vi "_PC_Spectrafilter get_tree_filter_data.vi"(8 "error in (no error)":errorcluster, 11 "file tree ref":refnum<vi>) -> (0 "error out":errorcluster, 2 "datas path":path[](array[path]))   [LabVIEW 2018]
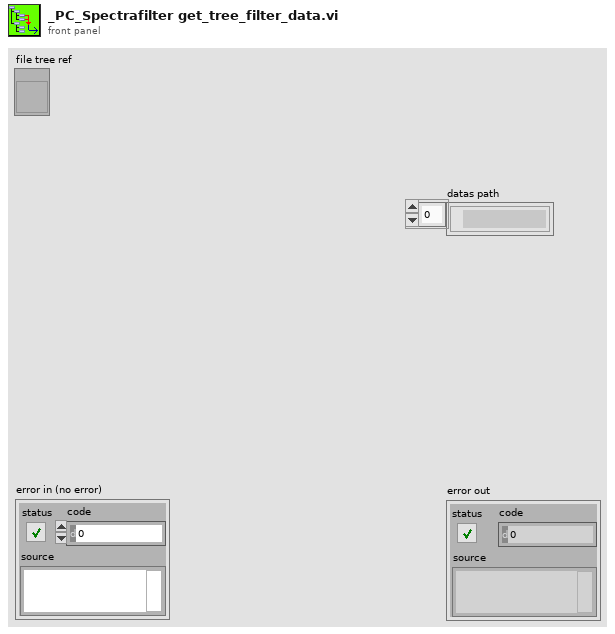
[diagram p1: front panel]
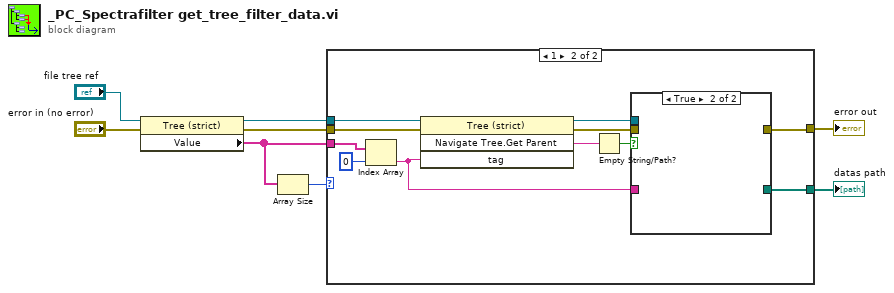
[diagram p0: block diagram]
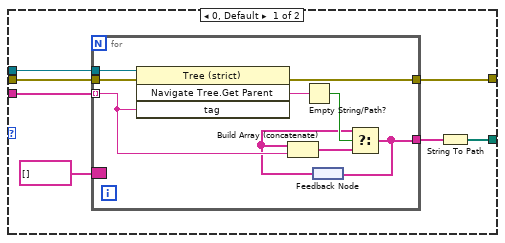
[diagram p2: hidden frame]
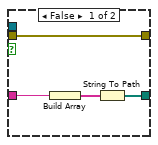
[diagram p3: hidden frame]
diagram:
  n1 = property class="Tree (strict)"(reference="file tree ref", error in="error in (no error)") -> (reference out=w8:refnum<vi>, error out=w3:errorcluster, "Value"=w7:string[])
  n2 = Array Size(array=w7) -> (size(s)=w6:i32)
  n3 = case shown="1" w6 {
    tunnel: w8 -> [w15 w35]
    tunnel: w7 -> [w14 w34]
    tunnel: [w11 w30] -> w1
    tunnel: w3 -> [w10 w27]
    tunnel: [w9 w25] -> w2
    frame 0, Default {
      n4 = for {
        tunnel: w15 -> [w24]
        tunnel: w14 -> [w21] mode=indexing
        tunnel: [w18] -> w12
        border: string[] [] -> [_]
        tunnel: w10 -> [w17]
        tunnel: [w16] -> w9
        n5 = invoke class="Tree (strict)" method="Navigate Tree.Get Parent"(reference=w24, error in=w17, "tag"=w21) -> (error out=w16:errorcluster, "Navigate Tree:Get Parent"=w23:string)  [unwired: 1 in, 2 out]
        n6 = Empty String/Path?(string/path=w23) -> (empty?=w22:bool)
        n7 = feedback #1() -> (w20:string[])
        n8 = Build Array (concatenate)(w20, w21) -> (w19:string[])
        n9 = Select(t=w20, s=w22, f=w19) -> (s? t:f=w18:string[])
        n10 = feedback-in #1(w18) -> ()
      }
      n11 = String To Path(string=w12) -> (path=w11:path[])
    }
    frame 1 {
      n12 = Index Array(array=w34, index=0) -> (element=w31:string)
      n13 = invoke class="Tree (strict)" method="Navigate Tree.Get Parent"(reference=w35, error in=w27, "tag"=w31) -> (reference out=w28:refnum<vi>, error out=w26:errorcluster, "Navigate Tree:Get Parent"=w32:string)  [unwired: 1 in, 1 out]
      n14 = Empty String/Path?(string/path=w32) -> (empty?=w29:bool)
      n15 = case shown="True" w29 {
        tunnel: w31 -> [w39 _]
        tunnel: [w37 _] -> w30
        tunnel: w28 -> [_ _]
        tunnel: w26 -> [w36 _]
        tunnel: [w36 _] -> w25
        frame False {
          n16 = Build Array(w39) -> (w38:string[])
          n17 = String To Path(string=w38) -> (path=w37:path[])
        }
        frame True {
        }
      }
    }
  }
  "error out" <- w2
  "datas path" <- w1
